vi "Scan action.vi"(6 "Index":i32, 7 "Comments":string, 8 "error in (no error)":errorcluster, 9 "Channels: AO":T2={"AO amp (V)"=[0.002, 0.002, 0.002, 0.002, 0.002, 0.002, 0.002, 0.002], "AO DC (V)"=[0.0, 0.0, 0.0, 0.0, 0.0, 0.0, 0.0, 0.0], "AO f (Hz)"=[15.1, 15.11, 15.12, 15.13, 15.14, 15.15, 15.16, 15.17], "AO phi (deg)"=[0.0, 10.0, 20.0, 30.0, 40.0, 50.0, 60.0, 70.0], "function"=[enum."Sine Wave", enum."Sine Wave", enum."Sine Wave", enum."Sine Wave", enum."Sine Wave", enum."Sine Wave", enum."Sine Wave", enum."Sine Wave"]} {"AO f (Hz)" min=0.001 max=10000.0; "AO DC (V)" format="%#_6p"; "AO amp (V)" format="%#_6p"}, 10 "Scan Name":T9=enum."DSA_Vamp", 11 "Scan Parameters":T1={"DAQ Channel"=2, "Label"="\nscaledVsg1=", "Start"=0.14, "End"=-0.060000000000000005, "Step"=-0.060000000000000005, "Rate"=-0.060000000000000005, "VISA resource name"="", "wait (ms)"=10000} {"Rate" format="%.2f"; "Step" format="%#_6p"; "End" format="%#_6p"; "Start" format="%#_6p"}) -> (0 "error out":errorcluster, 1 "Channels: AO":T2={"AO amp (V)"=[0.002, 0.002, 0.002, 0.002, 0.002, 0.002, 0.002, 0.002], "AO DC (V)"=[0.0, 0.0, 0.0, 0.0, 0.0, 0.0, 0.0, 0.0], "AO f (Hz)"=[15.1, 15.11, 15.12, 15.13, 15.14, 15.15, 15.16, 15.17], "AO phi (deg)"=[0.0, 10.0, 20.0, 30.0, 40.0, 50.0, 60.0, 70.0], "function"=[enum."Sine Wave", enum."Sine Wave", enum."Sine Wave", enum."Sine Wave", enum."Sine Wave", enum."Sine Wave", enum."Sine Wave", enum."Sine Wave"]} {"AO f (Hz)" min=0.001 max=10000.0; "AO DC (V)" format="%#_6p"; "AO amp (V)" format="%#_6p"}, 3 "Scan Parameters":T1={"DAQ Channel"=2, "Label"="\nscaledVsg1=", "Start"=0.14, "End"=-0.060000000000000005, "Step"=-0.060000000000000005, "Rate"=-0.060000000000000005, "VISA resource name"="", "wait (ms)"=10000} {"Rate" format="%.2f"; "Step" format="%#_6p"; "End" format="%#_6p"; "Start" format="%#_6p"}, 4 "Stop?":bool, 5 "Comments out":string)   [LabVIEW 2016, in "SweepControl.lvclass"]
uses:
  SweepControl.lvclass
  Typedefs/Enum - Action.ctl
  Typedefs/Cluster - ScanParamters.ctl
  <userlib>/LevyLab/Lockin-Multichannel/Typedefs/AO-cluster.ctl
  <userlib>/LevyLab/Lockin-Multichannel/Typedefs/AO_Amp-array.ctl
  <userlib>/LevyLab/Lockin-Multichannel/Typedefs/AO_DC-array.ctl
  <userlib>/LevyLab/Lockin-Multichannel/Typedefs/AO_f-array.ctl
  <userlib>/LevyLab/Lockin-Multichannel/Typedefs/AO_phi-array.ctl
  <userlib>/LevyLab/Lockin-Multichannel/Typedefs/Function-array.ctl
  <userlib>/LevyLab/Lockin-Multichannel/Typedefs/Function-enum.ctl
  <userlib>/LevyLab/Oxford 1820 API/Typedefs/Targets.ctl
panel:
  # "0"
  # "1"
  # "2"
  # "3"
  # "4"
  # "5"
  # "6"
  # "7"
  # "0"
  # "1"
  # "2"
  # "3"
  # "4"
  # "5"
  # "6"
  # "7"
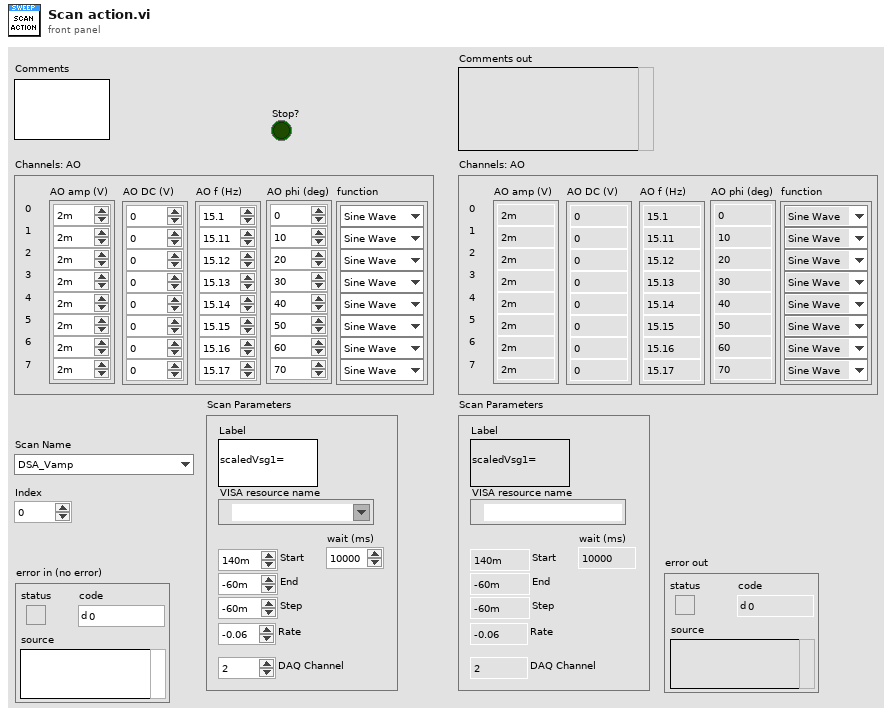
[diagram p1: front panel]
types:
  T1 = typedef "SweepControl.lvclass/Cluster - ScanParamters.ctl" = cluster{"DAQ Channel":i32, "Label":string, "Start":dbl, "End":dbl, "Step":dbl, "Rate":dbl, "VISA resource name":refnum<visa-resource-name>, "wait (ms)":u32}
  T2 = typedef "AO-cluster.ctl" = cluster{"AO amp (V)":T3, "AO DC (V)":T4, "AO f (Hz)":T5, "AO phi (deg)":T6, "function":T7}
  T3 = typedef "AO_Amp-array.ctl" = dbl[]
  T4 = typedef "AO_DC-array.ctl" = dbl[]
  T5 = typedef "AO_f-array.ctl" = dbl[]
  T6 = typedef "AO_phi-array.ctl" = dbl[]
  T7 = typedef "Function-array.ctl" = T8[]
  T8 = typedef "Function-enum.ctl" = enum16{"Sine Wave", "Triangle Wave", "Square Wave", "Sawtooth Wave"}
  T9 = typedef "SweepControl.lvclass/Enum - Action.ctl" = enum16{"OFF", "DSA_Vamp", "DSA_freq", "DSA_Vsg1", "DSA_Vsg2", "DSA_Vsg3", "DAQ_Vbg", "B_Field", "Humidity", "Temp", "MW_freq1", "MW_freq2", "MW_amplitude1", "MW_amplitude2"}
  T10 = typedef "Mercury-1820-API.lvlib/Targets.ctl" = cluster{"Target Field (T)":dbl, "Target Field Rate (T/min)":dbl}
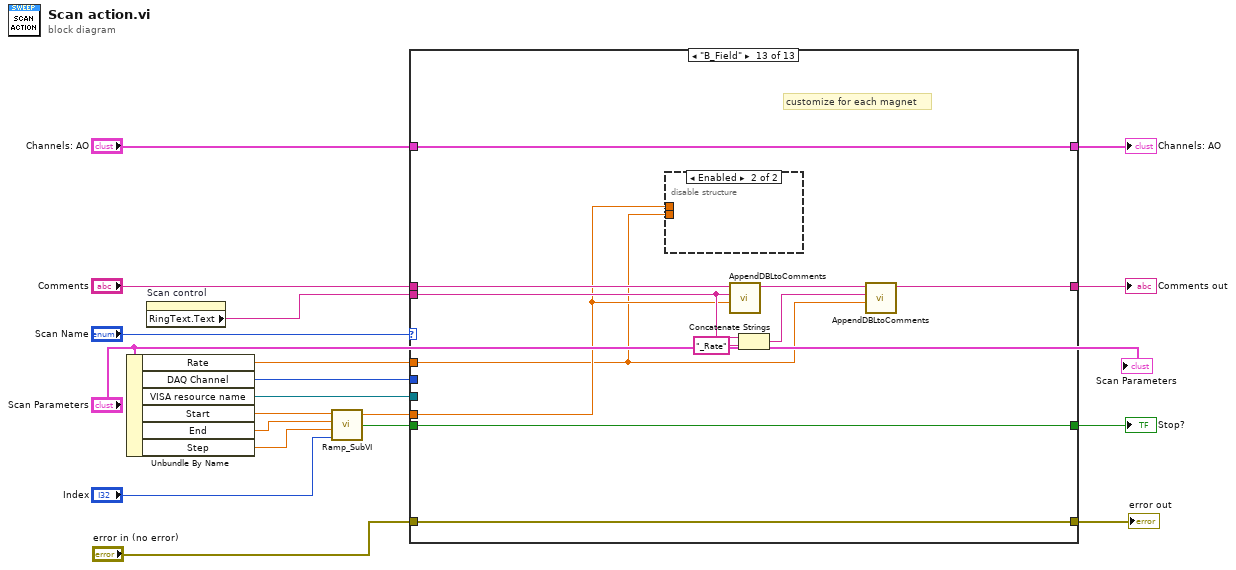
[diagram p0: block diagram]
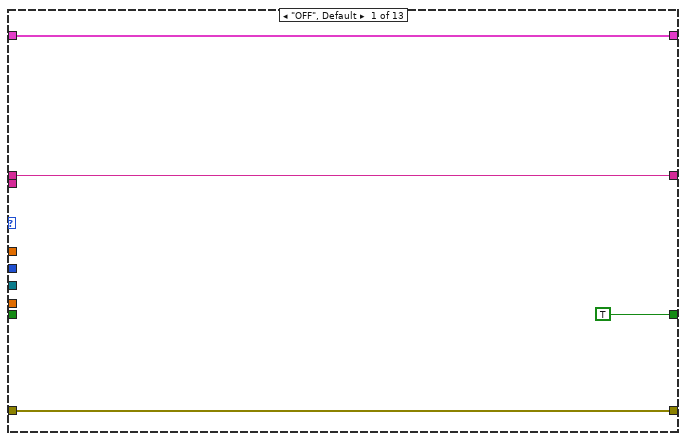
[diagram p2: hidden frame]
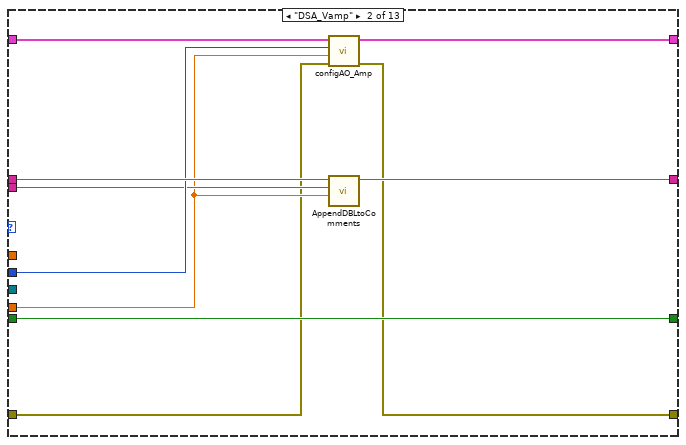
[diagram p3: hidden frame]
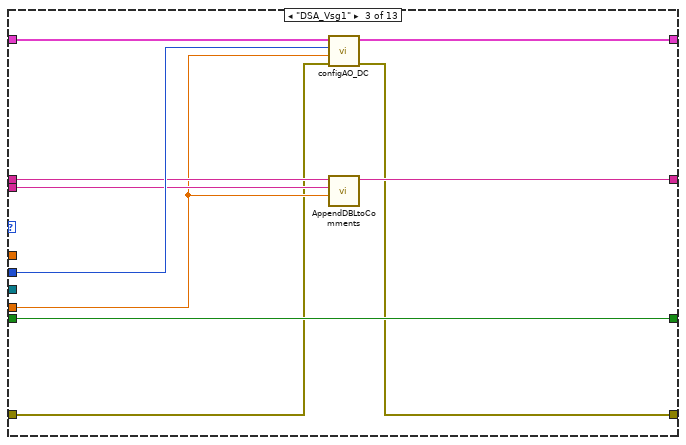
[diagram p4: hidden frame]
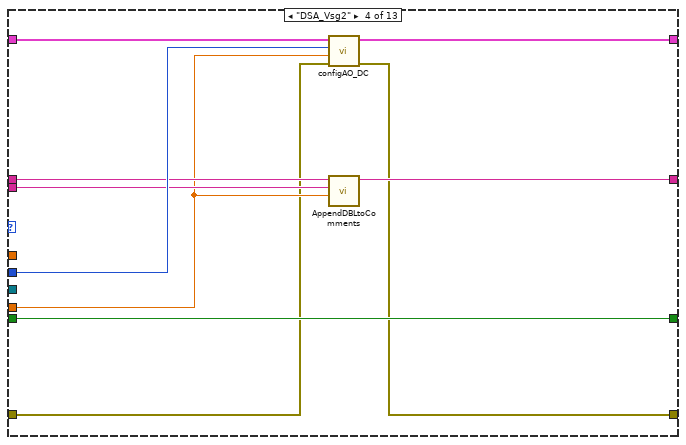
[diagram p5: hidden frame]
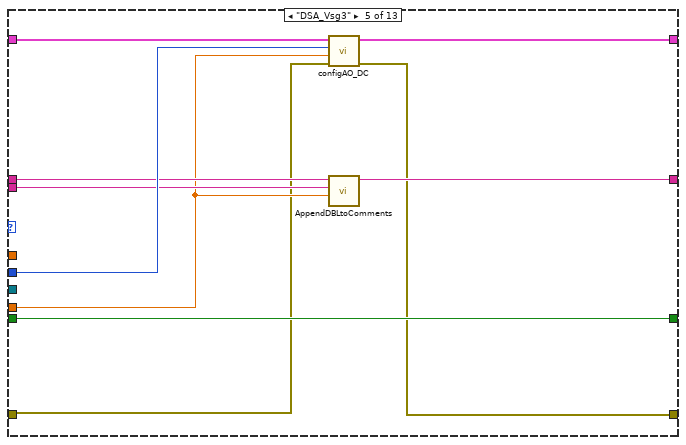
[diagram p6: hidden frame]
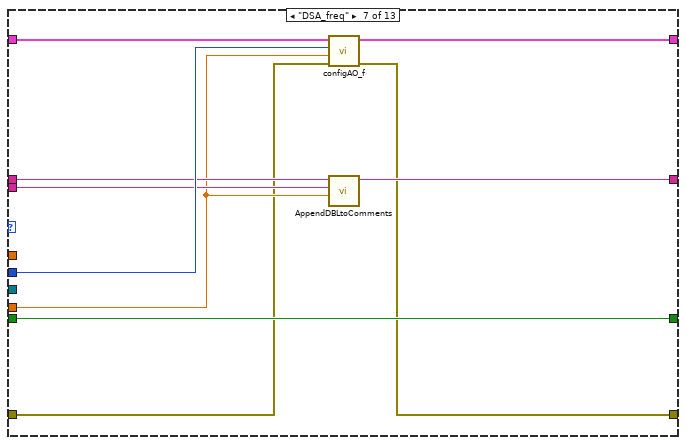
[diagram p8: hidden frame]
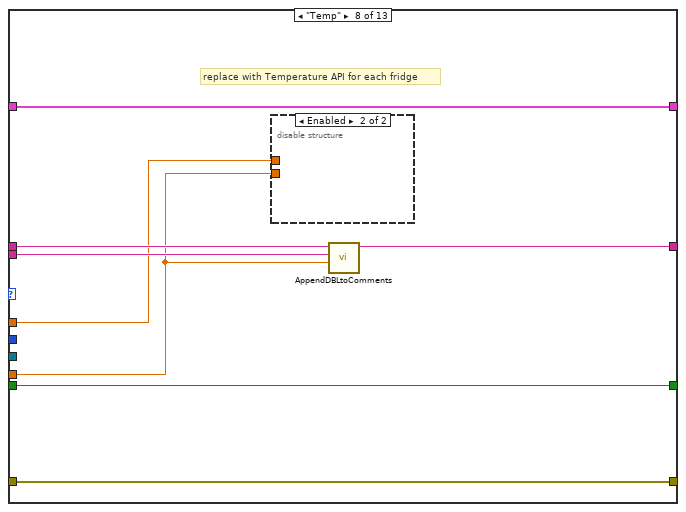
[diagram p9: hidden frame]
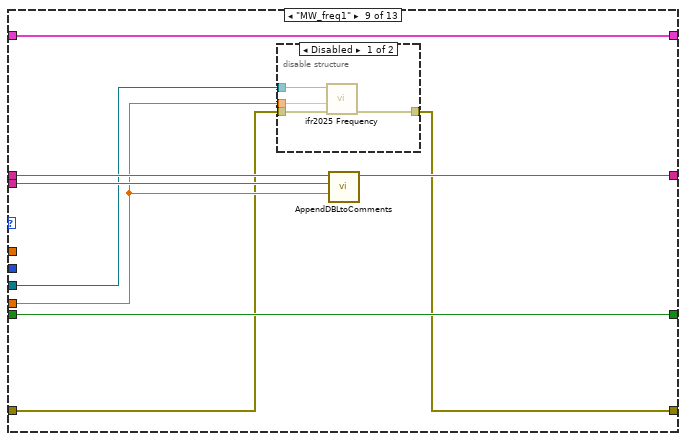
[diagram p11: hidden frame]
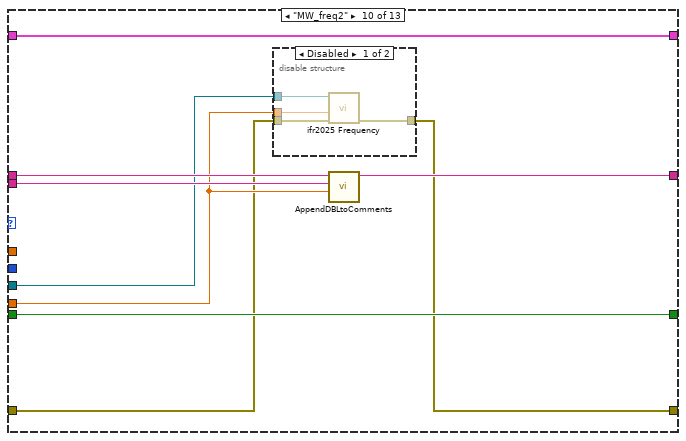
[diagram p13: hidden frame]
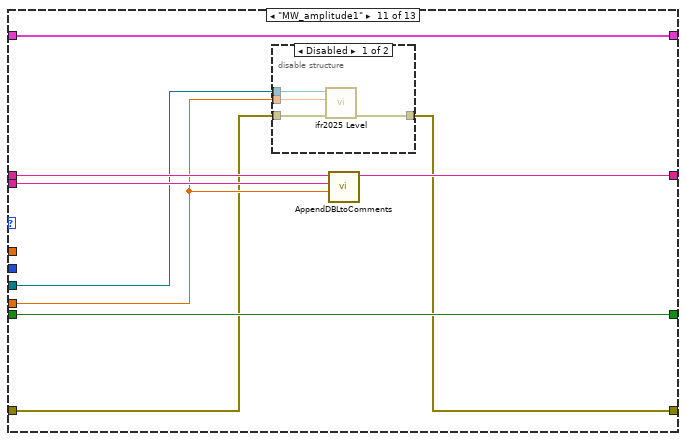
[diagram p15: hidden frame]
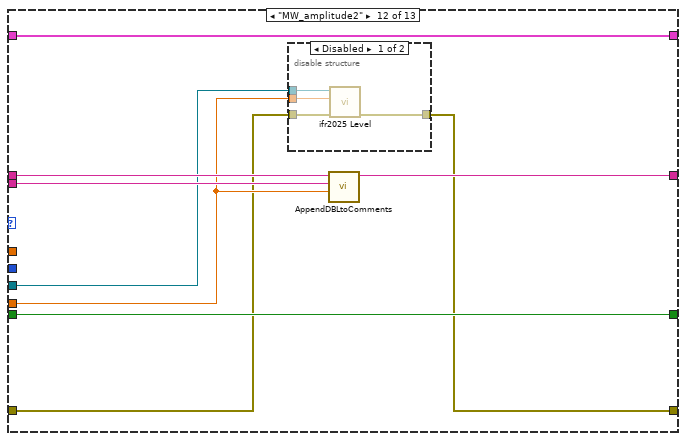
[diagram p17: hidden frame]
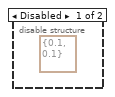
[diagram p19: hidden frame]
diagram:
  n1 = Unbundle By Name("Scan Parameters") -> ("Rate"=w12:dbl, "DAQ Channel"=w16:i32, "VISA resource name"=w4:refnum<visa-resource-name>, "Start"=w10:dbl, "End"=w9:dbl, "Step"=w8:dbl)
  n2 = property on="Scan control" class="Enum (strict)"() -> ("RingText.Text"=w11:string)  [unwired: 2 in, 2 out]
  n3 = call <userlib>:"Ramp_SubVI.vi"("index"="Index", "step"=w8, "end"=w9, "start"=w10) -> ("Stop?"=w6:bool, "Numeric"=w7:dbl)  [unwired: 1 in]
  n4 = case shown="\"B_Field\"" "Scan Name" {
    tunnel: w16 -> [_ w29 w41 w53 w63 _ w75 _ _ _ _ _ _]
    tunnel: "Comments" -> [w23 w33 w40 w50 w60 w66 w74 w84 w93 w106 w119 w132 w148]
    tunnel: w11 -> [_ w28 w38 w48 w58 _ w72 w82 w91 w104 w117 w130 w142]
    tunnel: [TRUE ("Stop?") w26 w36 w46 w56 w65 w70 w81 w90 w103 w116 w129 w147] -> w14
    tunnel: [w23 w32 w39 w49 w59 w66 w73 w83 w92 w105 w118 w131 w144] -> w13
    tunnel: "Channels: AO" -> [w21 w31 w43 w52 w62 w67 w77 w85 w94 w107 w120 w133 w146]
    tunnel: [w21 w30 w42 w51 w61 w67 w76 w85 w94 w107 w120 w133 w146] -> w18
    tunnel: w12 -> [_ _ _ _ _ _ _ w80 _ _ _ _ w139]
    tunnel: w7 -> [_ w27 w37 w47 w57 _ w71 w79 w89 w102 w115 w128 w140]
    tunnel: w6 -> [_ w26 w36 w46 w56 w65 w70 w81 w90 w103 w116 w129 w147]
    tunnel: w4 -> [_ _ _ _ _ _ _ _ w88 w101 w114 w127 _]
    tunnel: "error in (no error)" -> [w20 w25 w35 w45 w55 w64 w69 w78 w87 w100 w113 w126 w138]
    tunnel: [w20 w24 w34 w44 w54 w64 w68 w78 w86 w99 w112 w125 w138] -> w2
    frame "OFF", Default {
    }
    frame "DSA_Vamp" {
      n5 = call <userlib>:"configAO_Amp.vi"("error in (no error)"=w25, "new Amp (V)"=w27, "AO Channel"=w29, "Channels: AO"=w31) -> ("error out"=w24:errorcluster, "Channels: AO"=w30:T2)  [unwired: 6 in]
      n6 = call "AppendDBLtoComments.vi"("Numeric"=w27, "Label"=w28, "Comments in"=w33) -> ("Comments out"=w32:string)  [unwired: 8 in]
    }
    frame "DSA_Vsg1" {
      n7 = call <userlib>:"configAO_DC.vi"("error in (no error)"=w35, "new DC (V)"=w37, "AO Channel"=w41, "Channels: AO"=w43) -> ("error out"=w34:errorcluster, "Channels: AO"=w42:T2)  [unwired: 6 in]
      n8 = call "AppendDBLtoComments.vi"("Numeric"=w37, "Label"=w38, "Comments in"=w40) -> ("Comments out"=w39:string)  [unwired: 8 in]
    }
    frame "DSA_Vsg2" {
      n9 = call <userlib>:"configAO_DC.vi"("error in (no error)"=w45, "new DC (V)"=w47, "AO Channel"=w53, "Channels: AO"=w52) -> ("error out"=w44:errorcluster, "Channels: AO"=w51:T2)  [unwired: 6 in]
      n10 = call "AppendDBLtoComments.vi"("Numeric"=w47, "Label"=w48, "Comments in"=w50) -> ("Comments out"=w49:string)  [unwired: 8 in]
    }
    frame "DSA_Vsg3" {
      n11 = call <userlib>:"configAO_DC.vi"("error in (no error)"=w55, "new DC (V)"=w57, "AO Channel"=w63, "Channels: AO"=w62) -> ("error out"=w54:errorcluster, "Channels: AO"=w61:T2)  [unwired: 6 in]
      n12 = call "AppendDBLtoComments.vi"("Numeric"=w57, "Label"=w58, "Comments in"=w60) -> ("Comments out"=w59:string)  [unwired: 8 in]
    }
    frame "DAQ_Vbg" {
    }
    frame "DSA_freq" {
      n13 = call <userlib>:"configAO_f.vi"("error in (no error)"=w69, "new f (Hz)"=w71, "AO Channel"=w75, "Channels: AO"=w77) -> ("error out"=w68:errorcluster, "Channels: AO"=w76:T2)  [unwired: 6 in]
      n14 = call "AppendDBLtoComments.vi"("Numeric"=w71, "Label"=w72, "Comments in"=w74) -> ("Comments out"=w73:string)  [unwired: 8 in]
    }
    frame "Temp" {
      # "replace with Temperature API for each fridge"
      n15 = disable-structure shown="Enabled" {
        disable-tunnel: w80 -> [_ _]
        disable-tunnel: w79 -> [_ _]
        frame Disabled {
        }
        frame Enabled {
        }
      }
      n16 = call "AppendDBLtoComments.vi"("Numeric"=w79, "Label"=w82, "Comments in"=w84) -> ("Comments out"=w83:string)  [unwired: 8 in]
    }
    frame "MW_freq1" {
      n17 = disable-structure shown="Disabled" {
        disable-tunnel: w89 -> [w98 _]
        disable-tunnel: w88 -> [w97 _]
        disable-tunnel: w87 -> [w96 _]
        disable-tunnel: [w95 _] -> w86
        frame Disabled {
          n18 = call <instrlib>:"ifr2025 Frequency.vi"("error in (no error)"=w96, "Frequency (2.4E9)"=w98, "instrument handle"=w97) -> ("error out"=w95:errorcluster)  [unwired: 7 in, 1 out]
        }
        frame Enabled {
        }
      }
      n19 = call "AppendDBLtoComments.vi"("Numeric"=w89, "Label"=w91, "Comments in"=w93) -> ("Comments out"=w92:string)  [unwired: 8 in]
    }
    frame "MW_freq2" {
      n20 = disable-structure shown="Disabled" {
        disable-tunnel: w102 -> [w111 _]
        disable-tunnel: w101 -> [w110 _]
        disable-tunnel: w100 -> [w109 _]
        disable-tunnel: [w108 _] -> w99
        frame Disabled {
          n21 = call <instrlib>:"ifr2025 Frequency.vi"("error in (no error)"=w109, "Frequency (2.4E9)"=w111, "instrument handle"=w110) -> ("error out"=w108:errorcluster)  [unwired: 7 in, 1 out]
        }
        frame Enabled {
        }
      }
      n22 = call "AppendDBLtoComments.vi"("Numeric"=w102, "Label"=w104, "Comments in"=w106) -> ("Comments out"=w105:string)  [unwired: 8 in]
    }
    frame "MW_amplitude1" {
      n23 = disable-structure shown="Disabled" {
        disable-tunnel: w115 -> [w124 _]
        disable-tunnel: w114 -> [w123 _]
        disable-tunnel: w113 -> [w122 _]
        disable-tunnel: [w121 _] -> w112
        frame Disabled {
          n24 = call <instrlib>:"ifr2025 Level.vi"("error in (no error)"=w122, "RF Level (-137.0)"=w124, "instrument handle"=w123) -> ("error out"=w121:errorcluster)  [unwired: 7 in, 1 out]
        }
        frame Enabled {
        }
      }
      n25 = call "AppendDBLtoComments.vi"("Numeric"=w115, "Label"=w117, "Comments in"=w119) -> ("Comments out"=w118:string)  [unwired: 8 in]
    }
    frame "MW_amplitude2" {
      n26 = disable-structure shown="Disabled" {
        disable-tunnel: w128 -> [w137 _]
        disable-tunnel: w127 -> [w136 _]
        disable-tunnel: w126 -> [w135 _]
        disable-tunnel: [w134 _] -> w125
        frame Disabled {
          n27 = call <instrlib>:"ifr2025 Level.vi"("error in (no error)"=w135, "RF Level (-137.0)"=w137, "instrument handle"=w136) -> ("error out"=w134:errorcluster)  [unwired: 7 in, 1 out]
        }
        frame Enabled {
        }
      }
      n28 = call "AppendDBLtoComments.vi"("Numeric"=w128, "Label"=w130, "Comments in"=w132) -> ("Comments out"=w131:string)  [unwired: 8 in]
    }
    frame "B_Field" {
      # "customize for each magnet"
      n29 = disable-structure shown="Enabled" {
        disable-tunnel: w140 -> [_ _]
        disable-tunnel: w139 -> [_ _]
        frame Disabled {
          (unwired) T10 {"Target Field (T)"=0.1, "Target Field Rate (T/min)"=0.1} ("Mercury Targets")
        }
        frame Enabled {
        }
      }
      n30 = call "AppendDBLtoComments.vi"("Numeric"=w140, "Label"=w142, "Comments in"=w148) -> ("Comments out"=w145:string)  [unwired: 8 in]
      n31 = Concatenate Strings(w142, "_Rate" ("string")) -> (w141:string)
      n32 = call "AppendDBLtoComments.vi"("Numeric"=w139, "Label"=w141, "Comments in"=w145) -> ("Comments out"=w144:string)  [unwired: 8 in]
    }
  }
  "Comments out" <- w13
  "Stop?" <- w14
  "Channels: AO" <- w18
  "error out" <- w2
  "Scan Parameters" <- "Scan Parameters"
